vi "IRC-Pro_Test.vi"() -> ()   [LabVIEW 2019]
uses:
  <vilib>/myRIO/Common/Instrument Driver Framework/myRIO v1.0/UART/vis/myRIO v1.0 Close UART.vi
  <vilib>/myRIO/Common/Instrument Driver Framework/Utilities/vis/FPGA Ref Manager.vi
  <vilib>/myRIO/Common/Instrument Driver Framework/myRIO v1.0/myRIO v1.0 Reset FPGA.vi
  <vilib>/myRIO/Common/Instrument Driver Framework/myRIO v1.0/IRQ/vis/myRIO v1.0 IRQ Info FGV.vi
  <vilib>/myRIO/Common/Instrument Driver Framework/myRIO v1.0/IRQ/vis/myRIO v1.0 Timer IRQ Info FGV.vi
  <vilib>/myRIO/Common/Instrument Driver Framework/myRIO v1.0/IRQ/vis/myRIO v1.0 ISR Agent.vi
  <vilib>/myRIO/Instrument Drivers/Utilities/vis/Reset Index.vi
  <vilib>/myRIO/Common/Instrument Driver Framework/myRIO v1.0/Resource Manager/vis/myRIO v1.0 Block Write Resource Manager.vi
  <vilib>/myRIO/Instrument Drivers/Utilities/Utilities.lvlib
panel:
  out "Error Out":errorcluster
  in  "Error In":errorcluster
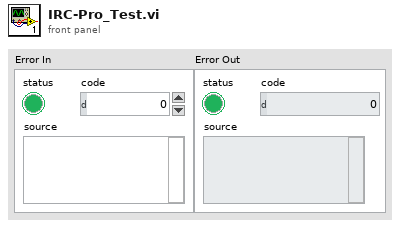
[diagram p1: front panel]
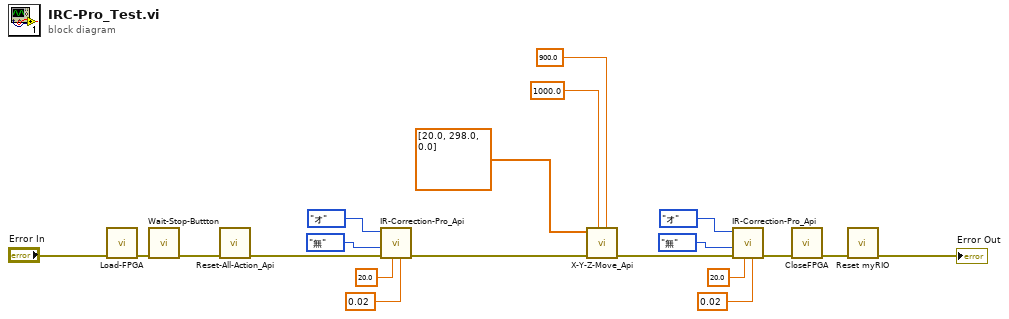
[diagram p0: block diagram]
diagram:
  n1 = call "Load-FPGA.vi"("Error In"="Error In") -> ("Error Out"=w20:errorcluster)  [unwired: 10 in]
  n2 = call "Wait-Stop-Buttton.vi"("Error In"=w20) -> ("Error Out"=w18:errorcluster)  [unwired: 10 in]
  n3 = call "Reset-All-Action_Api.vi"("Error In"=w18) -> ("Error Out"=w13:errorcluster)  [unwired: 8 in, 2 out]
  n4 = call "IR-Correction-Pro_Api.vi"("ExitRange"=0.02, "精準度"=20.0, "Error In"=w13, "副邊校正"=enum16{"前", "後", "オ", "右", "無"}."無", "主編校正"=enum16{"前", "後", "オ", "右", "無"}."オ") -> ("Error Out"=w7:errorcluster)  [unwired: 6 in]
  n5 = call "X-Y-Z-Move_Api.vi"("加速度"=900.0, "最高速"=1000.0, "Error In"=w7, "X-Y-Z移動"=dbl[] [20.0, 298.0, 0.0]) -> ("Error Out"=w1:errorcluster)  [unwired: 6 in, 1 out]
  n6 = call "IR-Correction-Pro_Api.vi"("ExitRange"=0.02, "精準度"=20.0, "Error In"=w1, "副邊校正"=enum16{"前", "後", "オ", "右", "無"}."無", "主編校正"=enum16{"前", "後", "オ", "右", "無"}."オ") -> ("Error Out"=w2:errorcluster)  [unwired: 6 in]
  n7 = call "CloseFPGA.vi"("Error In"=w2) -> ("Error Out"=w17:errorcluster)  [unwired: 10 in]
  n8 = call <vilib>:"Reset myRIO.vi"("error in (no error)"=w17) -> ("error out"=→"Error Out":errorcluster)  [unwired: 10 in]
